vi "Analysis.Build List of Unique Items, Str VariantAttributes.vi"(10 "Item In":string, 11 "List In":variant) -> (2 "Added":bool, 3 "List Out":variant, 5 "Index":i32)   [LabVIEW 2024]
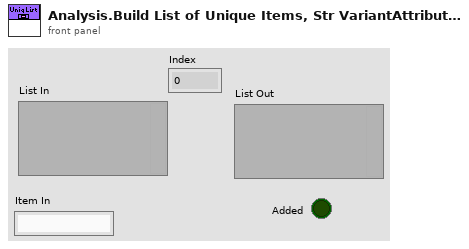
[diagram p1: front panel]
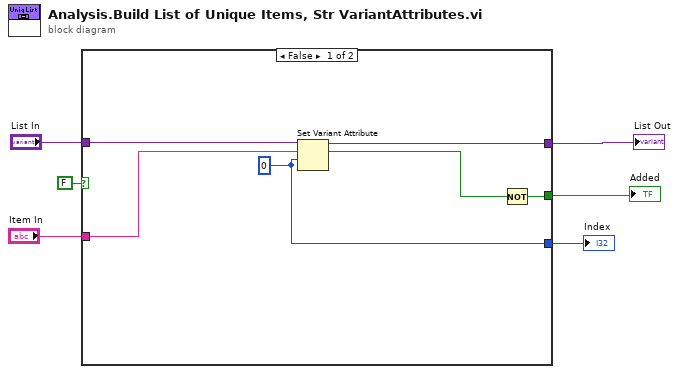
[diagram p0: block diagram]
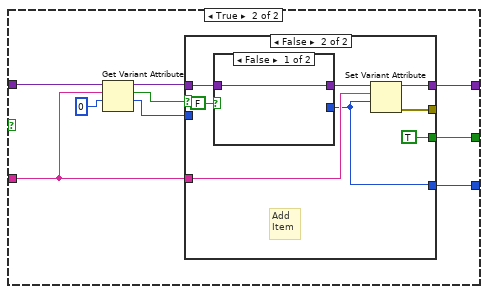
[diagram p2: hidden frame]
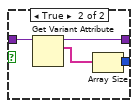
[diagram p4: hidden frame]
diagram:
  n1 = case shown="False" FALSE {
    tunnel: [w11 w21] -> w6
    tunnel: [w9 w20] -> w5
    tunnel: [w7 w19] -> w4
    tunnel: "List In" -> [w12 w18]
    tunnel: "Item In" -> [w10 w17]
    frame False {
      w7 = 0
      n2 = Set Variant Attribute(Variant=w12, name=w10, value=w7) -> (Variant out=w11:variant, replaced=w8:bool)  [unwired: 1 in, 1 out]
      n3 = Not(x=w8) -> (.not. x?=w9:bool)
    }
    frame True {
      n4 = Get Variant Attribute(Variant=w18, name=w17, default value (empty Variant)=0) -> (duplicate Variant=w16:variant, found=w15:bool, value=w13:i32)  [unwired: 1 in, 1 out]
      n5 = case shown="False" w15 {
        tunnel: w17 -> [_ w27]
        tunnel: w16 -> [w23 w30]
        tunnel: [w23 w29] -> w21
        tunnel: [_ TRUE] -> w20
        tunnel: [w22 w25] -> w19
        tunnel: w13 -> [w22 _]
        tunnel: [_ w26] -> _
        frame True {
          # "Skip"
        }
        frame False {
          # "Add\nItem"
          n6 = case shown="False" FALSE {
            tunnel: w30 -> [w32 w36]
            tunnel: [w32 w35] -> w28
            tunnel: [_ w34] -> w25
            frame False {
            }
            frame True {
              n7 = Get Variant Attribute(Variant=w36) -> (duplicate Variant=w35:variant, names=w33:string[])  [unwired: 3 in, 2 out]
              n8 = Array Size(array=w33) -> (size(s)=w34:i32)
            }
          }
          n9 = Set Variant Attribute(Variant=w28, name=w27, value=w25) -> (Variant out=w29:variant, error out=w26:errorcluster)  [unwired: 1 in, 1 out]
        }
      }
    }
  }
  "List Out" <- w6
  "Added" <- w5
  "Index" <- w4
